vi "Read Serial Port.vi"(8 "error in (no error)":errorcluster, 11 "NXP LPCXpresso54608 in":refnum<class "NXP LPCXpresso54608.lvclass">) -> (0 "error out":errorcluster, 2 "Serial Port":refnum<visa-resource-name>, 3 "NXP LPCXpresso54608 out":refnum<class "NXP LPCXpresso54608.lvclass">)   [LabVIEW 2020, in "NXP LPCXpresso54608.lvclass"]
uses:
  NXP LPCXpresso54608.lvclass
  NXP LPCXpresso54608.lvclass/NXP LPCXpresso54608.ctl
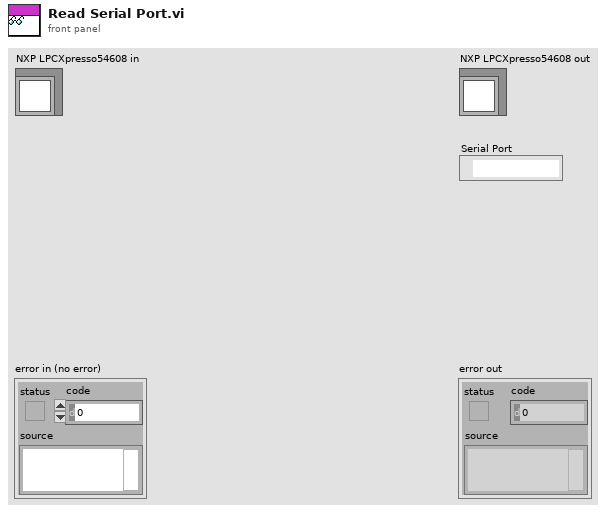
[diagram p1: front panel]
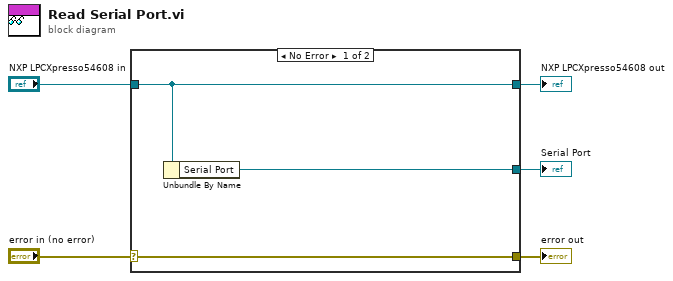
[diagram p0: block diagram]
diagram:
  n1 = case shown="No Error" "error in (no error)" {
    selector: "error in (no error)" -> [w8 w9]
    tunnel: [w8 w9] -> w4
    tunnel: [w7 w10] -> w2
    tunnel: "NXP LPCXpresso54608 in" -> [w7 w10]
    tunnel: [w6 _] -> w1
    frame No Error {
      n2 = Unbundle By Name(w7) -> ("Serial Port"=w6:refnum<visa-resource-name>)
    }
    frame Error {
    }
  }
  "error out" <- w4
  "NXP LPCXpresso54608 out" <- w2
  "Serial Port" <- w1
